vi "Time available for camera readout.vi"(9 "Trigger Jitter (ms)":dbl, 11 "Camera Settings":T1={"Exposure Time (ms)"=100.0, "Binning"=enum."2x2", "Scan Mode"=0, "Frames to Acquire"=1000.0, "Pixel Correction"=FALSE, "Frames to Skip"=0, "File Path"=path "", "Duty cycle"=0.0, "ALEX"=FALSE, "Shutter Enable"=[], "fluidics trigger frame"=0, "Bit Depth"=0, "Image Width (px)"=0, "Image Height (px)"=0, "Horizontal Offset (px)"=0, "Vertical Offset (px)"=0} {"fluidics trigger frame" max=60000 step=1; "Exposure Time (ms)" min=1.0 max=10000.0 step=1.0}) -> (1 "OK?":bool=TRUE, 2 "Min readout time (ms)":dbl=1000.0 format="%#_13g")   [LabVIEW 2023]
uses:
  Type Defs/Camera Settings.ctl
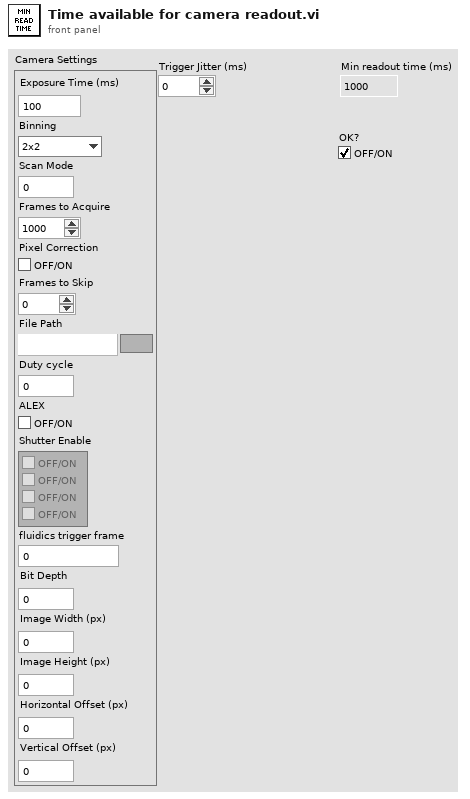
[diagram p1: front panel]
types:
  T1 = typedef "Camera Settings.ctl" = cluster{"Exposure Time (ms)":dbl, "Binning":enum16{"1x1", "2x2", "4x4"}, "Scan Mode":i32, "Frames to Acquire":dbl, "Pixel Correction":bool, "Frames to Skip":u32, "File Path":path, "Duty cycle":dbl, "ALEX":bool, "Shutter Enable":bool[], "fluidics trigger frame":u16, "Bit Depth":u16, "Image Width (px)":u16, "Image Height (px)":u16, "Horizontal Offset (px)":u16, "Vertical Offset (px)":u16}
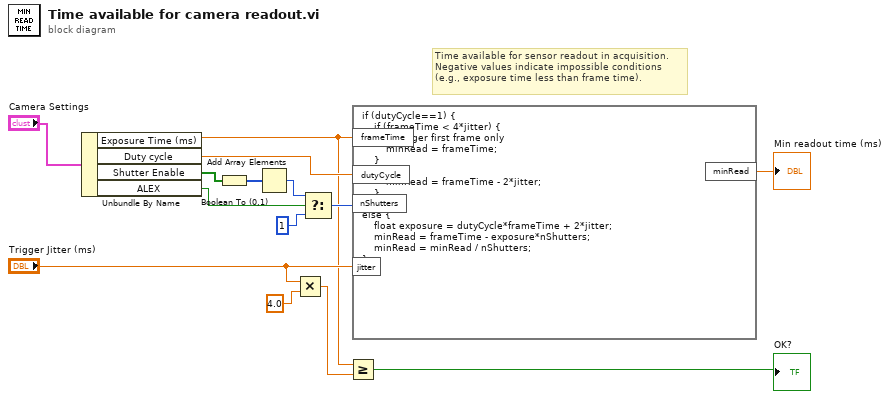
[diagram p0: block diagram]
diagram:
  # "Time available for sensor readout in acquisition.\nNegative values indicate impossible conditions\n(e.g., exposure time less than frame time)."
  n1 = Unbundle By Name("Camera Settings") -> ("Exposure Time (ms)"=w1:dbl, "Duty cycle"=w6:dbl, "Shutter Enable"=w13:bool[], "ALEX"=w10:bool)
  n2 = Boolean To (0,1)(Boolean=w13) -> (0, 1=w12:i16[])
  n3 = Add Array Elements(numeric array=w12) -> (sum=w11:i16)
  n4 = Multiply(x="Trigger Jitter (ms)", y=4.0) -> (x*y=w2:dbl)
  n5 = Select(t=w11, s=w10, f=i16 1) -> (s? t:f=w7:i16)
  n6 = Greater Or Equal?(x=w1, y=w2) -> (x >= y?=→"OK?":bool)
  n7 = formula code="if (dutyCycle==1) {\n    if (frameTime < 4*jitter) {\n        // trigger first frame only\n        minRead = frameTime;\n    }\n    else {\n        minRead = frameTime - 2*jitter;\n    }\n}\nelse {\n    float exposure = dutyCycle*frameTime + 2*jitter;\n    minRead = frameTime - exposure*nShutters;\n    minRead = minRead / nShutters;\n}"("frameTime"=w1, "dutyCycle"=w6, "nShutters"=w7, "jitter"="Trigger Jitter (ms)") -> ("minRead"=→"Min readout time (ms)":dbl)
